vi "PH_Cam_BaseClass.set configured.vi"(0 "i ref in":refnum<vi>, 2 "configured":bool, 5 "error in (no error)":errorcluster) -> (14 "i ref out":refnum<vi>, 19 "error out":errorcluster)   [LabVIEW 2014, in "PH_Cam_BaseClass.lvlib"]
doc: "This VI sets the camera attribute \"configured\" to own attributes and indicates it at the relevant GUI element."
uses:
  PH_Cam_BaseClass.lvlib
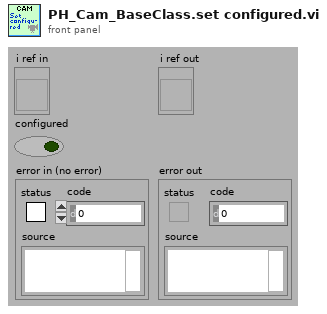
[diagram p1: front panel]
types:
  T1 = typedef "PH_Cam_BaseClass.lvlib/PH_Cam_BaseClass.i attribute.ctl" = cluster{"Gui Refs":T2, "Cam":cluster{"Source Notifier":refnum<notifier>, "Error":errorcluster, "Camera ID":string}, "Images":cluster{"Cam":T3, "Operation":T3, "PSDB":T3}, "Window Image":cluster{"Indicate Image":bool, "Window No.":i32, "Scale Facor":dbl, "Center Cross":bool, "Subtract Backgr":bool, "CoG":bool, "Color Palette":cluster{"Red":u8, "Green":u8, "Blue":u8}[], "Image On":bool}, "Default Prdc Int":i32, "Performance":cluster{"on":bool, "Timestamp Last Frame":i32}, "Histogram":cluster{"on":bool, "Mapping":bool}, "Save Image":cluster{"Save":bool, "File refnum":refnum<file>}, "Setting Service ID":i32, "Screen":cluster{"x-resolution":i16, "y-resolution":i16}, "On":bool, "Constructor finished":bool, "configured":bool}
  T2 = typedef "PH_Cam_BaseClass.lvlib/PH_Cam_BaseClass.GUI Refs.ctl" = cluster{"Frame Rate":refnum<vi>, "Get Frame Rate":refnum<vi>, "Show Image":refnum<vi>, "Get Histogram":refnum<vi>, "Mapping":refnum<vi>, "Histogram":refnum<vi>, "Center Cross":refnum<vi>, "Center of Gravity":refnum<vi>, "Scale Factor [%]":refnum<vi>, "Save Image":refnum<vi>, "Palette":refnum<vi>, "Subtract Background":refnum<vi>, "Cam Error":refnum<vi>, "On":refnum<vi>, "Cam List":refnum<vi>}
  T3 = typedef "IMAQ Image.ctl" = refnum<image>
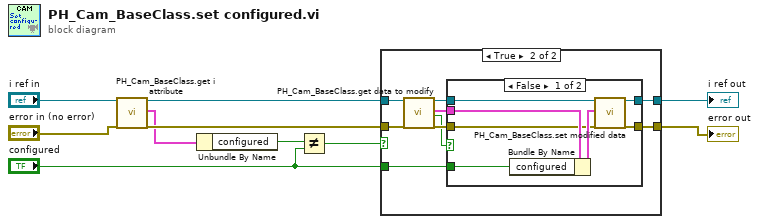
[diagram p0: block diagram]
diagram:
  n1 = call "PH_Cam_BaseClass.get i attribute.vi"("i ref in"="i ref in", "error in (no error)"="error in (no error)") -> ("i ref out"=w5:refnum<vi>, "i attribute"=w4:T1, "error out"=w7:errorcluster)  [unwired: 15 in]
  n2 = Unbundle By Name(w4) -> ("configured"=w3:bool)
  n3 = Not Equal?(x=w3, y="configured") -> (x != y?=w1:bool)
  n4 = case shown="True" w1 {
    tunnel: [w11 w21] -> w10
    tunnel: [w12 w20] -> w9
    tunnel: w7 -> [w11 w15]
    tunnel: w5 -> [w12 w14]
    tunnel: "configured" -> [_ w13]
    frame False {
    }
    frame True {
      n5 = call "PH_Cam_BaseClass.get data to modify.vi"("i ref in"=w14, "error in (no error)"=w15) -> ("i ref out"=w18:refnum<vi>, "i attribute"=w16:T1, "timed out"=w17:bool, "error out"=w19:errorcluster)  [unwired: 14 in]
      n6 = case shown="False" w17 {
        tunnel: w19 -> [w22 w29]
        tunnel: [w28 w29] -> w21
        tunnel: w18 -> [w27 w30]
        tunnel: [w26 w30] -> w20
        tunnel: w16 -> [w24 _]
        tunnel: w13 -> [w23 _]
        frame False {
          n7 = Bundle By Name(cluster=w24, "configured"=w23) -> (w25:T1)
          n8 = call "PH_Cam_BaseClass.set modified data.vi"("i ref in"=w27, "i attribute"=w25, "error in (no error)"=w22) -> ("i ref out"=w26:refnum<vi>, "error out"=w28:errorcluster)  [unwired: 15 in]
        }
        frame True {
        }
      }
    }
  }
  "error out" <- w10
  "i ref out" <- w9
